vi "Format Tables String.vi"(0 "Header":string[](array[string]), 5 "Data Table":string[][](array[string])) -> (4 "spreadsheet string":string)   [LabVIEW 2010]
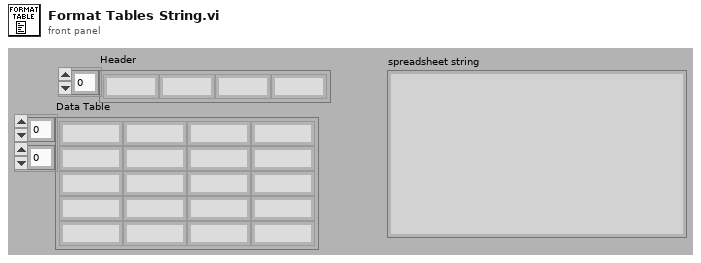
[diagram p1: front panel]
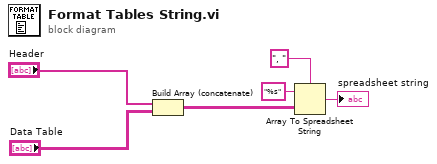
[diagram p0: block diagram]
diagram:
  n1 = Build Array (concatenate)("Header", "Data Table") -> (w5:string[][])
  n2 = Array To Spreadsheet String(delimiter (Tab)=", ", array=w5, 3:"%s" ("format string")) -> (spreadsheet string=→"spreadsheet string":string)
